vi "GLB_compteurs.vi"() -> ()   [LabVIEW 2014, in "PLS Digital Control.lvlib"]
uses:
  PLS Digital Control.lvlib
panel:
  in  "total":cluster{"c0":dbl, "c1":dbl, "c2":dbl, "c3":dbl}
  in  "live":cluster{"c0":dbl, "c1":dbl, "c2":dbl, "c3":dbl}
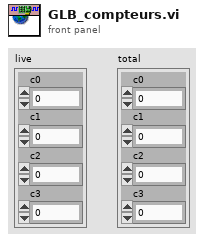
[diagram p1: front panel]
diagram:
